vi "test.vi"   [LabVIEW 2014]
uses:
  <vilib>/Utility/file.llb/Write To Spreadsheet File (DBL).vi
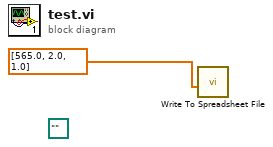
[diagram p0: block diagram]
diagram:
  (unwired) path ""
  n1 = call-poly <vilib>:"Write To Spreadsheet File.vi"("1D data"=dbl[] [565.0, 2.0, 1.0]) -> ()  [unwired: 7 in, 1 out]
